vi "Variable@Delete__Parameter.vi"(1 "ParamterIn":string) -> (0 "ParamterOut":string)   [LabVIEW 2020]
panel:
  in  "Section":string(combo)
  in  "ParameterName":string(combo)
  in  "Confirm":bool
  # "Variable@Del $Variable(,$Section)"
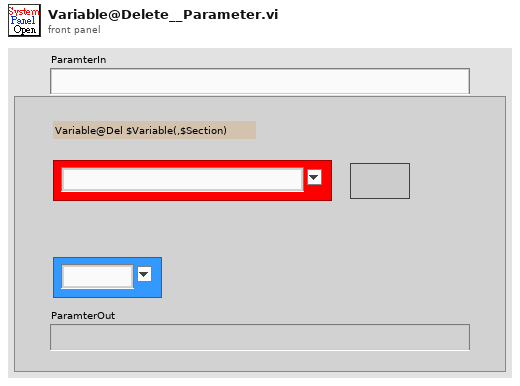
[diagram p1: front panel]
types:
  T1 = enum16{"Get", "Init", "Set", "Delete", "GetElement", "Inc", "Dec"}
  T2 = enum16{"Get", "Init", "Set", "Delete", "GetElement", "Inc", "Dec", "ReName"}
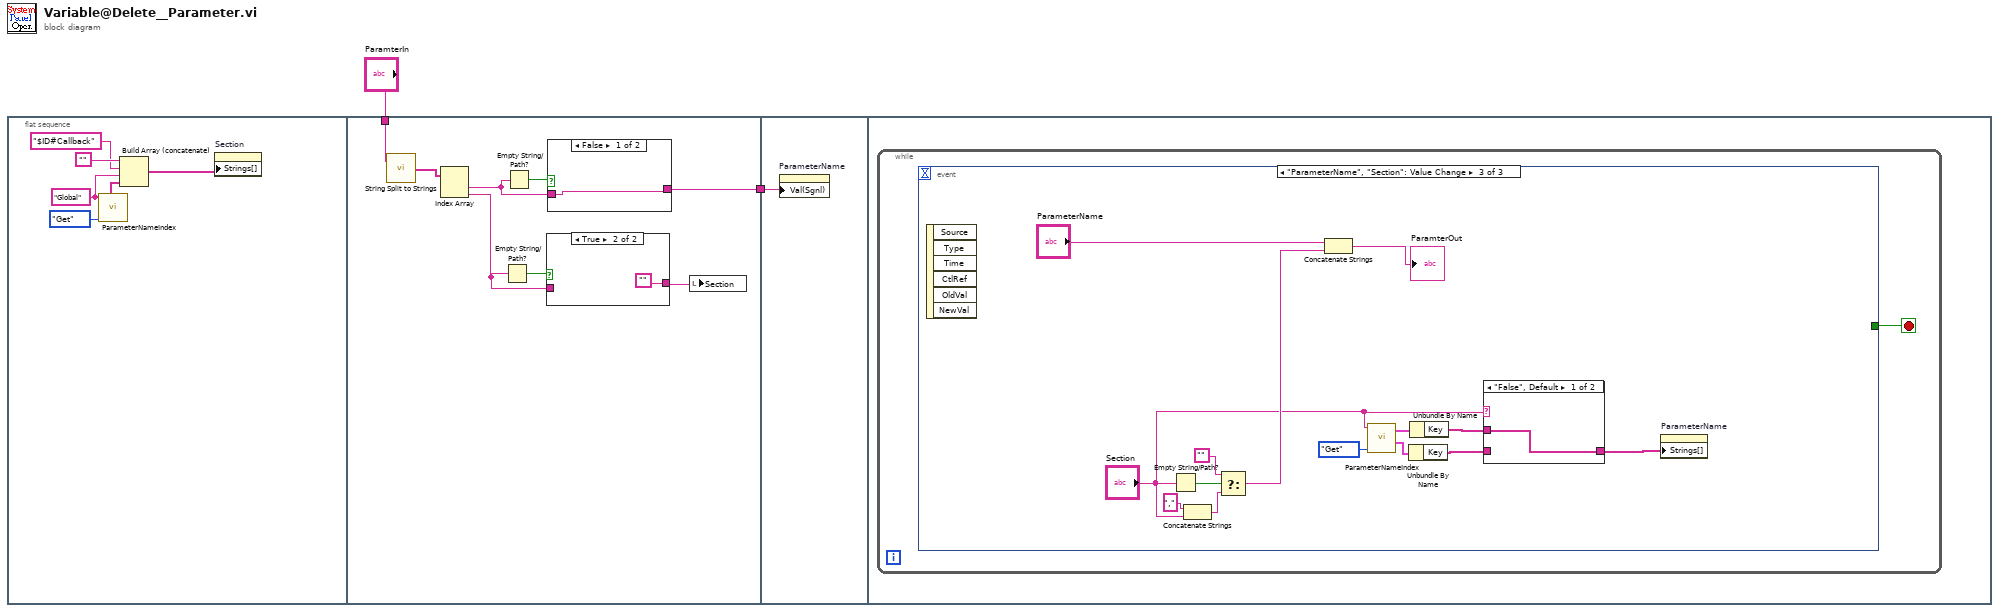
[diagram p0: block diagram]
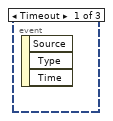
[diagram p4: hidden frame]
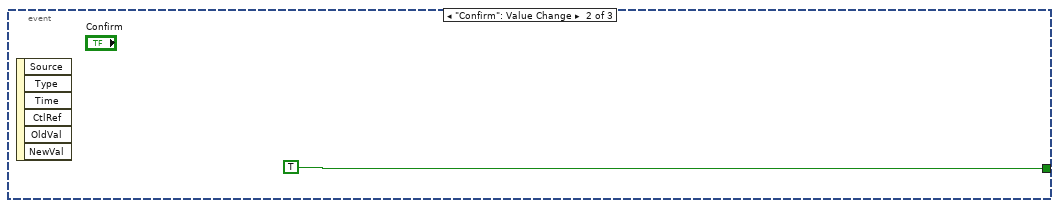
[diagram p5: hidden frame]
diagram:
  n1 = flat-sequence {
    tunnel: "ParamterIn" -> [w13]
    tunnel: [w14] -> w1
    tunnel: w1 -> [w21]
    frame #0 {
      w5 = "Global" ("VariableSection")
      n2 = call "ParameterNameIndex.vi"("OP"=T1."Get", "VariableSection"=w5) -> ("SectionList"=w6:string[])  [unwired: 3 in, 6 out]
      n3 = Build Array (concatenate)("", "$ID#Callback" ("VariableSection"), w5, w6) -> (w4:string[])
      n4 = property on="Section" class="CmbBox"("Strings[]"=w4) -> ()  [unwired: 2 in, 2 out]
    }
    frame #1 {
      n5 = call "String Split to Strings.vi"("String"=w13) -> ("Array"=w12:string[])  [unwired: 1 in]
      n6 = Index Array(array=w12) -> (element #1=w11:string, element #2=w10:string)  [unwired: 2 in]
      n7 = Empty String/Path?(string/path=w10) -> (empty?=w15:bool)
      n8 = Empty String/Path?(string/path=w11) -> (empty?=w16:bool)
      n9 = case shown="True" w15 {
        tunnel: w10 -> [w17 _]
        tunnel: [w17 ""] -> w9
        frame False {
        }
        frame True {
        }
      }
      n10 = case shown="False" w16 {
        tunnel: w11 -> [w19 w20]
        tunnel: [w19 w20] -> w14
        frame False {
        }
        frame True {
        }
      }
      n11 = local write "Section"(w9) -> ()
    }
    frame #2 {
      n12 = property on="ParameterName" class="CmbBox"("Val(Sgnl)"=w21) -> ()  [unwired: 2 in, 2 out]
    }
    frame #3 {
      n13 = while {
        stop <- w22 stop-if-true
        n14 = event shown="[2] \"ParameterName\", \"Section\": Value Change" {
          selector: _ -> [_ _ _]
          dyn-events: _ -> [_ _ _]
          timeout: _ -> [_ _ _]
          tunnel: [_ TRUE _] -> w22
          event Timeout {
            n15 = event-data() -> ()  [unwired: 1 in, 3 out]
          }
          event "Confirm": Value Change {
            n16 = event-data() -> ()  [unwired: 1 in, 6 out]
          }
          event "ParameterName", "Section": Value Change {
            n17 = event-data() -> ()  [unwired: 1 in, 6 out]
            n18 = Empty String/Path?(string/path="Section") -> (empty?=w33:bool)
            n19 = Concatenate Strings("," ("string"), "Section") -> (w34:string)
            n20 = Select(t="", s=w33, f=w34) -> (s? t:f=w32:string)
            n21 = Concatenate Strings("ParameterName", w32) -> (→"ParamterOut":string)
            n22 = call "ParameterNameIndex.vi"("OP"=T2."Get", "VariableSection"="Section") -> ("GlobalKeyValue"=w28:cluster{"Key":string[], "Value":string[]}, "SectionKeyValue"=w27:cluster{"Key":string[], "Value":string[]})  [unwired: 3 in, 5 out]
            n23 = Unbundle By Name(w28) -> ("Key"=w29:string[])
            n24 = Unbundle By Name(w27) -> ("Key"=w30:string[])
            n25 = case shown="\"False\", Default" "Section" {
              tunnel: w29 -> [_ w39]
              tunnel: [w38 w39] -> w24
              tunnel: w30 -> [w38 _]
              frame "False", Default {
              }
              frame "", "Global" {
              }
            }
            n26 = property on="ParameterName" class="CmbBox"("Strings[]"=w24) -> ()  [unwired: 2 in, 2 out]
          }
        }
      }
    }
  }
